vi "Configure Temperature (Thermocouple).vi"(0 "VISA resource name":refnum<visa-resource-name>, 1 "Unit (1: Celsius)":i32(ring)=1 items=["Kelvin", "Celsius", "Fahrenheit"], 2 "Thermocouple Type (3: K)":i32(ring)=3 items=["B", "E", "J", "K", "N", "R", "S", "T"], 5 "Reference Junction Type (1: Internal)":i32(ring)=1 items=["Simulated", "Internal", "External"], 9 "Channel List(\"\")":string, 11 "error in (no error)":errorcluster, 12 "Simulated Reference Temperature (0)":dbl) -> (4 "VISA resource name out":refnum<visa-resource-name>, 15 "error out":errorcluster)   [LabVIEW 2019, in "Keithley DMM6500 DAQ6500 Series.lvlib"]
doc: "Configures the temperature thremal sensor with thermocouple."
uses:
  Keithley DMM6500 DAQ6500 Series.lvlib
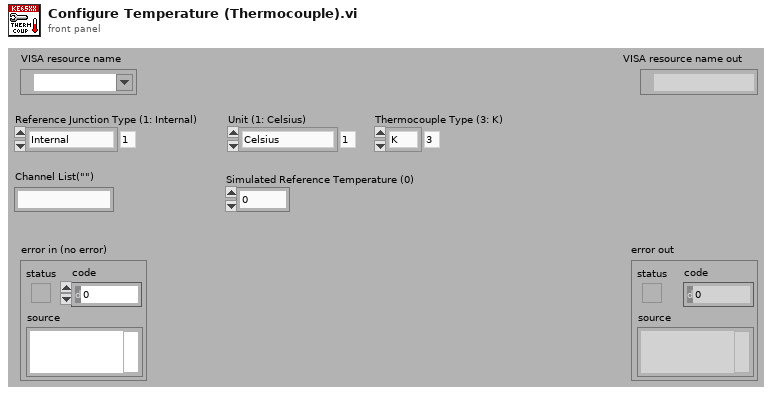
[diagram p1: front panel]
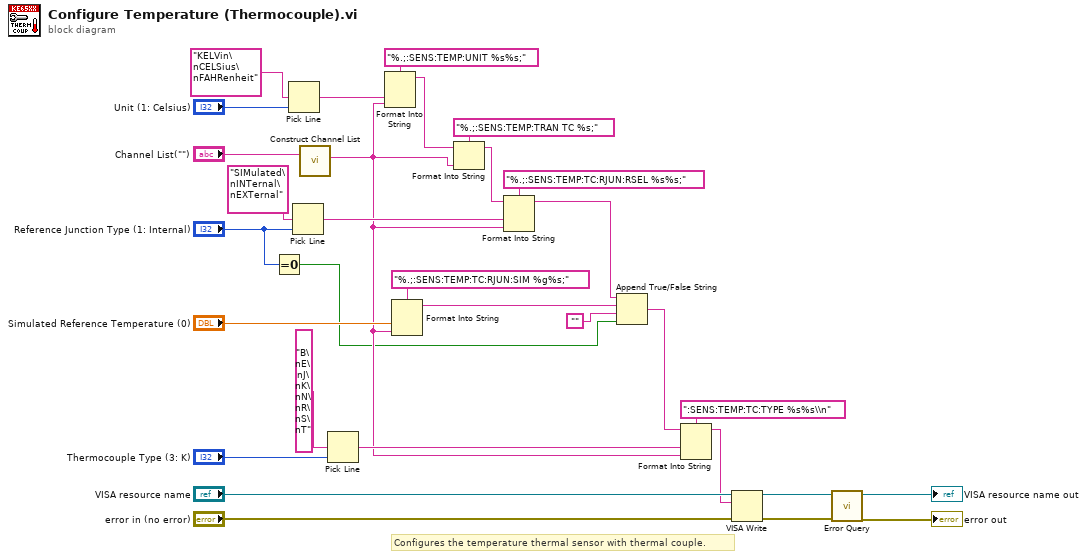
[diagram p0: block diagram]
diagram:
  # "Configures the temperature thermal sensor with thermal couple."
  n1 = Equal To 0?(x="Reference Junction Type (1: Internal)") -> (x = 0?=w2:bool)
  n2 = Pick Line(multi-line string="KELVin\nCELSius\nFAHRenheit", line index="Unit (1: Celsius)") -> (output string=w18:string)  [unwired: 1 in]
  n3 = Pick Line(multi-line string="SIMulated\nINTernal\nEXTernal", line index="Reference Junction Type (1: Internal)") -> (output string=w14:string)  [unwired: 1 in]
  n4 = call "Construct Channel List.vi"("Channel List"="Channel List(\"\")") -> ("Channel List String"=w3:string)  [unwired: 2 in]
  n5 = Pick Line(multi-line string="B\nE\nJ\nK\nN\nR\nS\nT", line index="Thermocouple Type (3: K)") -> (output string=w11:string)  [unwired: 1 in]
  n6 = Format Into String(format string="%.;:SENS:TEMP:UNIT %s%s;", w18, w3) -> (resulting string=w17:string)  [unwired: 2 in, 1 out]
  n7 = Format Into String(format string="%.;:SENS:TEMP:TC:RJUN:SIM %g%s;", "Simulated Reference Temperature (0)", w3) -> (resulting string=w5:string)  [unwired: 2 in, 1 out]
  n8 = Format Into String(format string="%.;:SENS:TEMP:TRAN TC %s;", initial string=w17, w3) -> (resulting string=w9:string)  [unwired: 1 in, 1 out]
  n9 = Format Into String(format string="%.;:SENS:TEMP:TC:RJUN:RSEL %s%s;", initial string=w9, w14, w3) -> (resulting string=w6:string)  [unwired: 1 in, 1 out]
  n10 = Append True/False String(1:w2, 2:"", 3:w5, 4:w6) -> (0:w7:string)
  n11 = Format Into String(format string=":SENS:TEMP:TC:TYPE %s%s\\n", initial string=w7, w11, w3) -> (resulting string=w8:string)  [unwired: 1 in, 1 out]
  n12 = VISA Write(VISA resource name="VISA resource name", write buffer=w8, error in (no error)="error in (no error)") -> (VISA resource name out=w25:refnum<visa-resource-name>, error out=w24:errorcluster)  [unwired: 1 out]
  n13 = call "Error Query.vi"("error in (no error)"=w24, "VISA resource name"=w25) -> ("error out"=→"error out":errorcluster, "VISA resource name out"=→"VISA resource name out":refnum<visa-resource-name>)  [unwired: 6 in, 2 out]
